vi "Setup Arcadia_lv2015.vi"(11 "error in (no error)":errorcluster) -> (2 "LabVIEW Versions Present":string[](array[string]))   [LabVIEW 2015]
uses:
  <vilib>/nisyscfg/Get Installed Components.vi
  <vilib>/nisyscfg/Close (System).vi
  <vilib>/nisyscfg/nisyscfg.lvlib
panel:
  out "?":u8(slide) scale=0.0..100.0
  out "error out":errorcluster
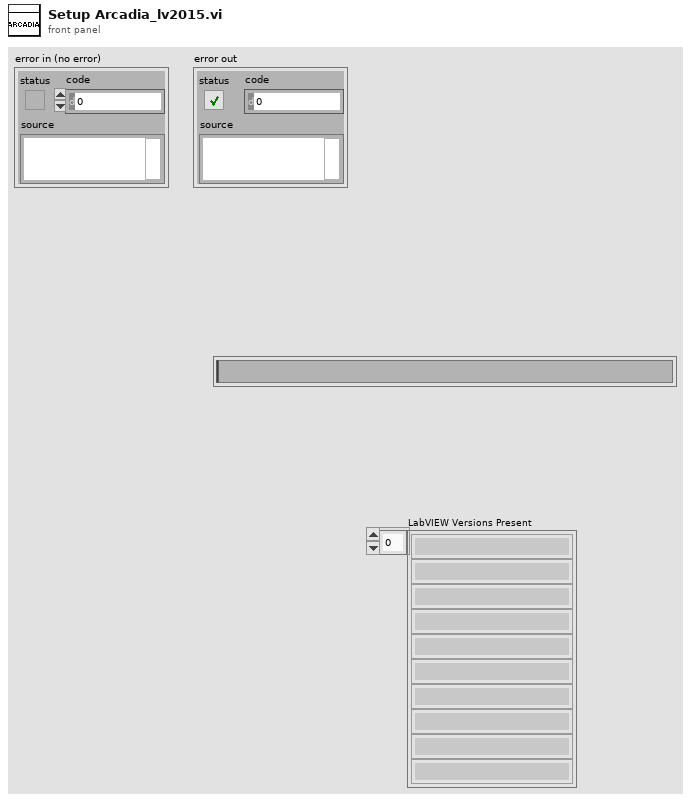
[diagram p1: front panel]
types:
  T1 = typedef "nisyscfg.lvlib/Software 1.2.ctl" = cluster{"title":string, "description":string, "ID":string, "version":string, "component type":T2}
  T2 = typedef "nisyscfg.lvlib/Component Type.ctl" = u32
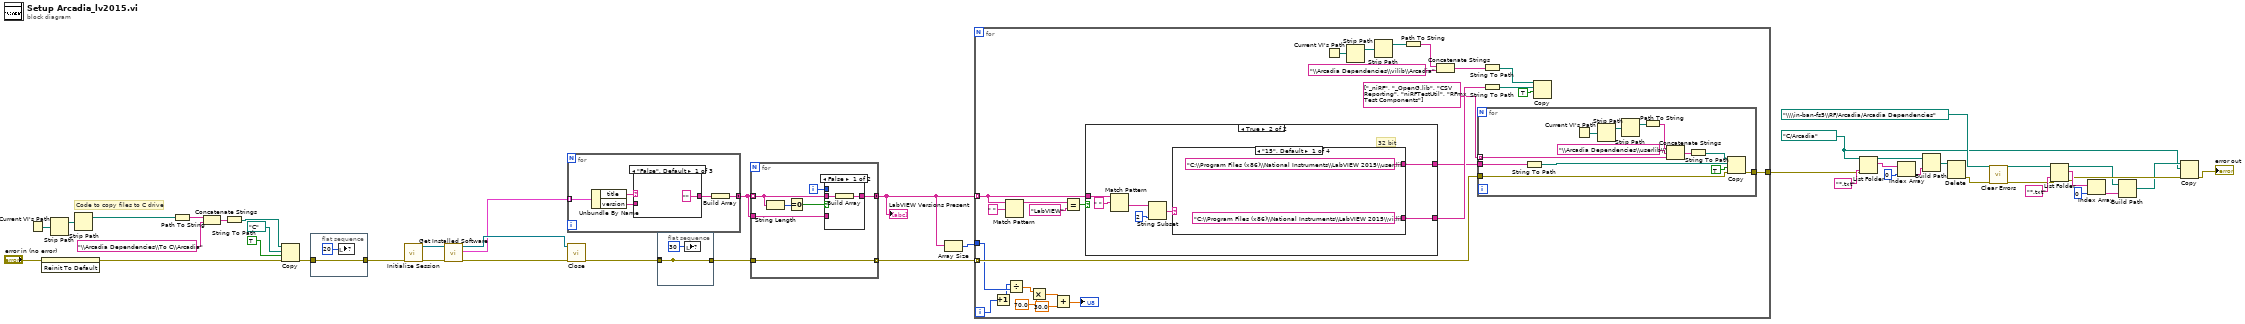
[diagram p0: block diagram]
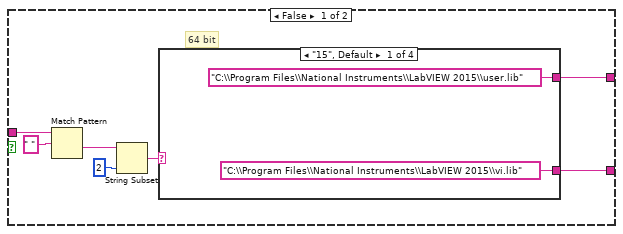
[diagram p2: hidden frame]
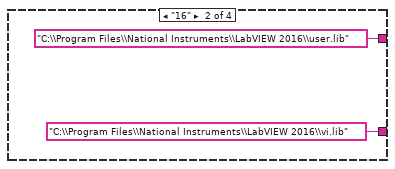
[diagram p3: hidden frame]
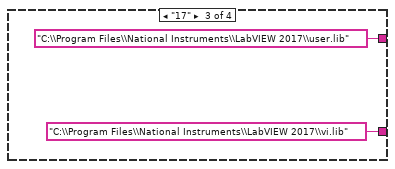
[diagram p4: hidden frame]
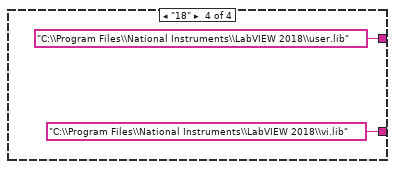
[diagram p5: hidden frame]
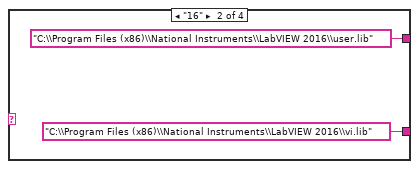
[diagram p6: hidden frame]
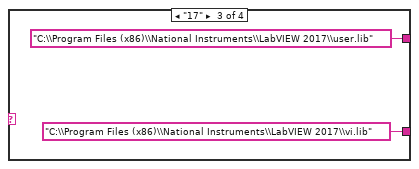
[diagram p7: hidden frame]
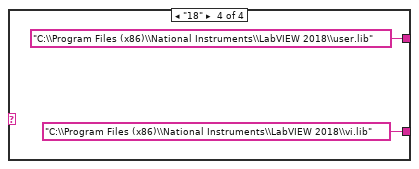
[diagram p8: hidden frame]
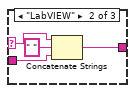
[diagram p10: hidden frame]
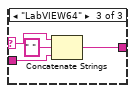
[diagram p11: hidden frame]
diagram:
  w6 = path "C:/Arcadia" ("path")
  # "Code to copy files to C drive"
  n1 = Current VI's Path() -> (path=w31:path)
  n2 = invoke class="Slide (strict)" method="Reinit To Default"(error in="error in (no error)") -> (error out=w25:errorcluster)  [unwired: 2 in, 2 out]
  n3 = Strip Path(path=w31) -> (stripped path=w34:path)  [unwired: 1 out]
  n4 = Strip Path(path=w34) -> (stripped path=w35:path)  [unwired: 1 out]
  n5 = Path To String(path=w35) -> (string=w32:string)
  n6 = Concatenate Strings(w32, "\\Arcadia Dependencies\\To C\\Arcadia" ("string")) -> (w30:string)
  n7 = String To Path(string=w30) -> (path=w29:path)
  n8 = Copy(8:w25, 9:TRUE ("overwrite (F)"), 10:path "C:/" ("target path (use dialog)"), 11:w29) -> (0:w23:errorcluster)  [unwired: 1 in, 2 out]
  n9 = flat-sequence {
    tunnel: w23 -> [w44]
    tunnel: [w44] -> w1
    frame #0 {
      n10 = local write item#3(u8 20) -> ()
    }
  }
  n11 = call <vilib>:"Initialize Session.vi"("error in (no error)"=w1) -> ("error out"=w42:errorcluster, "Session out"=w43:refnum<k21>)  [unwired: 9 in]
  n12 = call-poly <vilib>:"Get Installed Software.vi"("error in (no error)"=w42, "Session in"=w43) -> ("error out"=w41:errorcluster, "Software Components"=w39:T1[], "Session out"=w40:refnum<k21>)  [unwired: 7 in]
  n13 = for {
    tunnel: w39 -> [w50] mode=indexing
    tunnel: [w46] -> w38 mode=concatenating
    n14 = Unbundle By Name(w50) -> ("title"=w48:string, "version"=w49:string)
    n15 = case shown="\"False\", Default" w48 {
      selector: w48 -> [_ w55 w57]
      tunnel: w49 -> [_ w53 w58]
      tunnel: ["" w52 w56] -> w47
      frame "False", Default {
      }
      frame "LabVIEW" {
        n16 = Concatenate Strings(w55, " " ("string"), w53) -> (w52:string)
      }
      frame "LabVIEW64" {
        n17 = Concatenate Strings(w57, " " ("string"), w58) -> (w56:string)
      }
    }
    n18 = Build Array(w47) -> (w46:string[])
  }
  n19 = call-poly <vilib>:"Close.vi"("error in (no error)"=w41, "Session in"=w40) -> ("error out"=w22:errorcluster)  [unwired: 9 in]
  n20 = flat-sequence {
    tunnel: [w60] -> _
    tunnel: [w60] -> w21
    tunnel: w22 -> [w60]
    frame #0 {
      n21 = local write item#3(u8 30) -> ()
    }
  }
  n22 = for {
    tunnel: w38 -> [w64] mode=indexing
    tunnel: w38 -> [w65]
    tunnel: [w63] -> w27 mode=concatenating
    tunnel: w21 -> [w62]
    tunnel: [w62] -> w28 mode=indexing
    i -> [w66]
    n23 = String Length(string=w64) -> (length=w68:i32)
    n24 = Equal To 0?(x=w68) -> (x = 0?=w67:bool)
    n25 = case shown="False" w67 {
      tunnel: w66 -> [_ _]
      tunnel: w65 -> [_ _]
      tunnel: w64 -> [w70 _]
      tunnel: [w69 _] -> w63
      frame False {
        n26 = Build Array(w70) -> (w69:string[])
      }
      frame True {
      }
    }
  }
  "LabVIEW Versions Present" <- w27
  n27 = Array Size(array=w27) -> (size(s)=w26:i32)
  n28 = for {
    tunnel: w27 -> [w93] mode=indexing
    tunnel: [w80] -> w3
    tunnel: w28 -> [w79] mode=indexing
    tunnel: w26 -> [w78]
    i -> [w72]
    n29 = Increment(x=w72) -> (x+1=w71:i32)
    n30 = Match Pattern(string=w93, regular expression=" ") -> (before substring=w94:string)  [unwired: 1 in, 3 out]
    n31 = Divide(x=w71, y=w78) -> (x/y=w77:dbl)
    n32 = Multiply(x=w77, y=70.0 ("x")) -> (x*y=w75:dbl)
    n33 = Add(x=w75, y=30.0) -> (x+y=→"?":dbl)
    n34 = Equal?(x=w94, y="LabVIEW") -> (x = y?=w95:bool)
    n35 = case shown="True" w95 {
      tunnel: w93 -> [w116 w131]
      tunnel: [w112 w127] -> w83
      tunnel: [w111 w126] -> w81
      frame False {
        # "64 bit"
        n36 = Match Pattern(string=w116, regular expression=" ") -> (after substring=w115:string)  [unwired: 1 in, 3 out]
        n37 = String Subset(string=w115, length (rest)=2 ("length (rest)")) -> (substring=w113:string)  [unwired: 1 in]
        n38 = case shown="\"15\", Default" w113 {
          tunnel: ["C:\\Program Files\\National Instruments\\LabVIEW 2015\\vi.lib" "C:\\Program Files\\National Instruments\\LabVIEW 2016\\vi.lib" "C:\\Program Files\\National Instruments\\LabVIEW 2017\\vi.lib" "C:\\Program Files\\National Instruments\\LabVIEW 2018\\vi.lib"] -> w112
          tunnel: ["C:\\Program Files\\National Instruments\\LabVIEW 2015\\user.lib" "C:\\Program Files\\National Instruments\\LabVIEW 2016\\user.lib" "C:\\Program Files\\National Instruments\\LabVIEW 2017\\user.lib" "C:\\Program Files\\National Instruments\\LabVIEW 2018\\user.lib"] -> w111
          frame "15", Default {
          }
          frame "16" {
          }
          frame "17" {
          }
          frame "18" {
          }
        }
      }
      frame True {
        # "32 bit"
        n39 = Match Pattern(string=w131, regular expression=" ") -> (after substring=w129:string)  [unwired: 1 in, 3 out]
        n40 = String Subset(string=w129, length (rest)=2 ("length (rest)")) -> (substring=w128:string)  [unwired: 1 in]
        n41 = case shown="\"15\", Default" w128 {
          tunnel: ["C:\\Program Files (x86)\\National Instruments\\LabVIEW 2015\\vi.lib" "C:\\Program Files (x86)\\National Instruments\\LabVIEW 2016\\vi.lib" "C:\\Program Files (x86)\\National Instruments\\LabVIEW 2017\\vi.lib" "C:\\Program Files (x86)\\National Instruments\\LabVIEW 2018\\vi.lib"] -> w127
          tunnel: ["C:\\Program Files (x86)\\National Instruments\\LabVIEW 2015\\user.lib" "C:\\Program Files (x86)\\National Instruments\\LabVIEW 2016\\user.lib" "C:\\Program Files (x86)\\National Instruments\\LabVIEW 2017\\user.lib" "C:\\Program Files (x86)\\National Instruments\\LabVIEW 2018\\user.lib"] -> w126
          frame "15", Default {
          }
          frame "16" {
          }
          frame "17" {
          }
          frame "18" {
          }
        }
      }
    }
    n42 = Current VI's Path() -> (path=w87:path)
    n43 = Strip Path(path=w87) -> (stripped path=w90:path)  [unwired: 1 out]
    n44 = Strip Path(path=w90) -> (stripped path=w91:path)  [unwired: 1 out]
    n45 = Path To String(path=w91) -> (string=w88:string)
    n46 = Concatenate Strings(w88, "\\Arcadia Dependencies\\vilib\\Arcadia" ("string")) -> (w86:string)
    n47 = for {
      tunnel: string[] ["_niRF", "_OpenG.lib", "CSV Reporting", "niRFTestUtil", "RFmx Test Components"] -> [w101] mode=indexing
      tunnel: w81 -> [w100]
      tunnel: [w99] -> w80
      tunnel: w79 -> [w98]
      n48 = String To Path(string=w100) -> (path=w102:path)
      n49 = Current VI's Path() -> (path=w110:path)
      n50 = Strip Path(path=w110) -> (stripped path=w107:path)  [unwired: 1 out]
      n51 = Strip Path(path=w107) -> (stripped path=w106:path)  [unwired: 1 out]
      n52 = Path To String(path=w106) -> (string=w109:string)
      n53 = Concatenate Strings(w109, "\\Arcadia Dependencies\\userlib\\" ("string"), w101) -> (w104:string)
      n54 = String To Path(string=w104) -> (path=w103:path)
      n55 = Copy(8:w98, 9:TRUE ("overwrite (F)"), 10:w102, 11:w103) -> (0:w99:errorcluster)  [unwired: 1 in, 2 out]
    }
    n56 = String To Path(string=w86) -> (path=w85:path)
    n57 = String To Path(string=w83) -> (path=w84:path)
    n58 = Copy(9:TRUE ("overwrite (F)"), 10:w84, 11:w85) -> ()  [unwired: 2 in, 3 out]
  }
  n59 = List Folder(path=w6, pattern="*.txt", error in=w3) -> (path out=w19:path, filenames=w18:string[])  [unwired: 1 in, 2 out]
  n60 = Index Array(array=w18, index=0) -> (element=w16:string)
  n61 = Build Path(base path=w19, name or relative path=w16) -> (appended path=w15:path)
  n62 = Delete(path (use dialog)=w15) -> (error out=w5:errorcluster)  [unwired: 4 in, 2 out]
  n63 = call <vilib>:"Clear Errors.vi"("error in (no error)"=w5) -> ("error out"=w4:errorcluster)  [unwired: 5 in, 1 out]
  n64 = List Folder(path=path "\\\\in-ban-fs5\\RF/Arcadia/Arcadia Dependencies", pattern="*.txt", error in=w4) -> (path out=w8:path, filenames=w11:string[], error out=w10:errorcluster)  [unwired: 1 in, 1 out]
  n65 = Index Array(array=w11, index=0) -> (element=w9:string)
  n66 = Build Path(base path=w8, name or relative path=w9) -> (appended path=w7:path)
  n67 = Copy(8:w10, 10:w6, 11:w7) -> (0:→"error out":errorcluster)  [unwired: 2 in, 2 out]
